vi "soliton-lock-error signal monitor real time.vi"() -> ()   [LabVIEW 2011]
panel:
  out "Meter":dbl(knob)=0.9830155860081771 scale=-0.5..0.5
  out "data":dbl=0.2882122313383335
  in  "stop (F)":bool
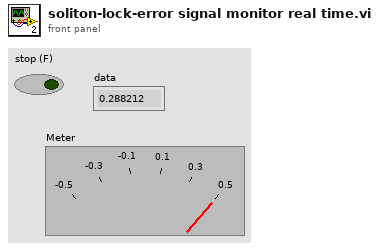
[diagram p1: front panel]
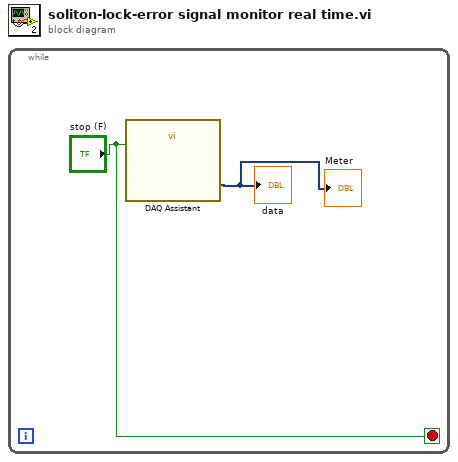
[diagram p0: block diagram]
diagram:
  n1 = while {
    stop <- "stop (F)" stop-if-true
    n2 = call "DAQ Assistant"("stop (T)"="stop (F)") -> ("data"=→"data" →"Meter":dynamicdata)  [unwired: 16 in, 2 out]
  }
